vi "Default Error File Path.vi"(8 "error in (no error)":errorcluster) -> (0 "error out":errorcluster, 3 "Default Path":path)   [LabVIEW 2018]
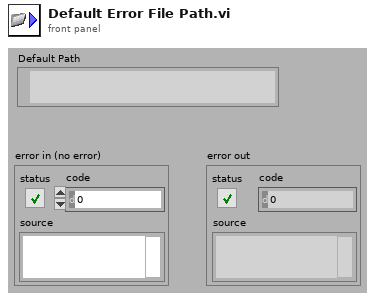
[diagram p1: front panel]
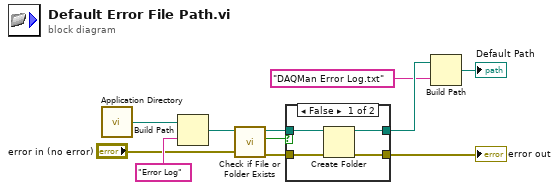
[diagram p0: block diagram]
diagram:
  n1 = call <vilib>:"Application Directory.vi"() -> ("Application Directory"=w10:path)
  n2 = Build Path(base path=w10, name or relative path="Error Log") -> (appended path=w6:path)
  n3 = call <vilib>:"Check if File or Folder Exists.vi"("error in (no error)"="error in (no error)", "path"=w6) -> ("error out"=w7:errorcluster, "file or folder exists?"=w8:bool, "dup path"=w9:path)  [unwired: 7 in]
  n4 = case shown="False" w8 {
    tunnel: w9 -> [w15 w16]
    tunnel: w7 -> [w14 w17]
    tunnel: [w13 w17] -> w5
    tunnel: [w12 w16] -> w3
    frame False {
      n5 = Create Folder(path (use dialog)=w15, error in=w14) -> (created path=w12:path, error out=w13:errorcluster)  [unwired: 1 in, 1 out]
    }
    frame True {
    }
  }
  "error out" <- w5
  n6 = Build Path(base path=w3, name or relative path="DAQMan Error Log.txt") -> (appended path=→"Default Path":path)
